vi "Cleanup.vi"(0 "Library Builder in":refnum<class "Library Builder.lvclass">, 5 "Remove 64-bit Project?":bool=TRUE, 11 "error in (no error)":errorcluster) -> (4 "Library Builder out":refnum<class "Library Builder.lvclass">, 6 "Project Path":path, 8 "Working Directory":path, 10 "Version":u32, 15 "error out":errorcluster)   [LabVIEW 2020, in "Library Builder.lvclass"]
uses:
  Library Builder.lvclass
  Library Builder.lvclass/Library Builder.ctl
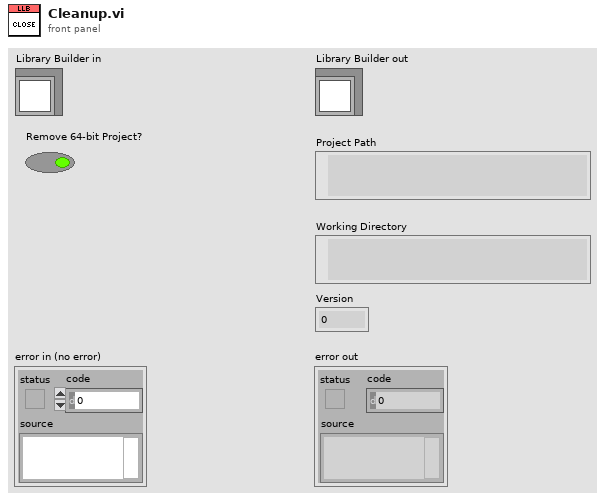
[diagram p1: front panel]
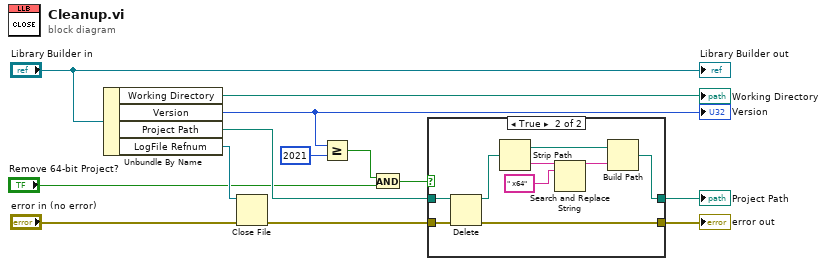
[diagram p0: block diagram]
diagram:
  n1 = Unbundle By Name("Library Builder in") -> ("Working Directory"=→"Working Directory":path, "Version"=w8:u32, "Project Path"=w6:path, "LogFile Refnum"=w11:refnum<file>)
  "Version" <- w8
  n2 = Close File(refnum=w11, error in="error in (no error)") -> (error out=w7:errorcluster)  [unwired: 1 out]
  n3 = Greater Or Equal?(x=w8, y=u32 2021 ("Version")) -> (x >= y?=w2:bool)
  n4 = And(x=w2, y="Remove 64-bit Project?") -> (x .and. y?=w1:bool)
  n5 = case shown="True" w1 {
    tunnel: w7 -> [w14 w24]
    tunnel: w6 -> [w15 w22]
    tunnel: [w15 w17] -> w4
    tunnel: [w14 w16] -> w5
    frame False {
    }
    frame True {
      n6 = Delete(path (use dialog)=w22, error in=w24) -> (deleted path=w23:path, error out=w16:errorcluster)  [unwired: 3 in, 1 out]
      n7 = Strip Path(path=w23) -> (stripped path=w21:path, name=w20:string)
      n8 = Search and Replace String(input string=w20, search string=" x64") -> (result string=w18:string)  [unwired: 6 in, 3 out]
      n9 = Build Path(base path=w21, name or relative path=w18) -> (appended path=w17:path)
    }
  }
  "error out" <- w5
  "Project Path" <- w4
  "Library Builder out" <- "Library Builder in"
